vi "search for available lvclass files.vi"(6 "Folders to Exclude":string[](array[string]), 8 "error in":errorcluster, 11 "Plugin Search Paths":path[](array[path])) -> (0 "error out":errorcluster, 3 "discovered classes":path[](array[path]))   [LabVIEW 2013, in "class discovery singleton.lvlib"]
doc: "Finds all lvclass files, even inside llb and lvlibp files. Removes any in a folder titled \"\\builds\\\"."
uses:
  class discovery singleton.lvlib
  <vilib>/Utility/LVLibp/NI_PackedLibraryUtility.lvlib
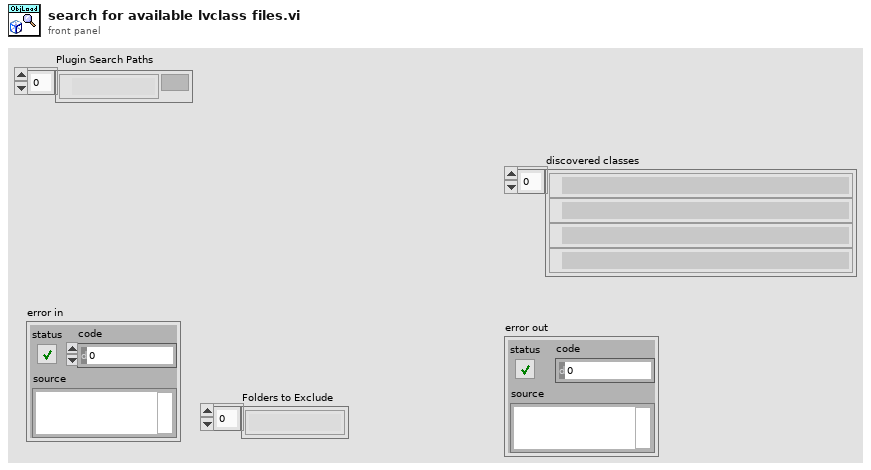
[diagram p1: front panel]
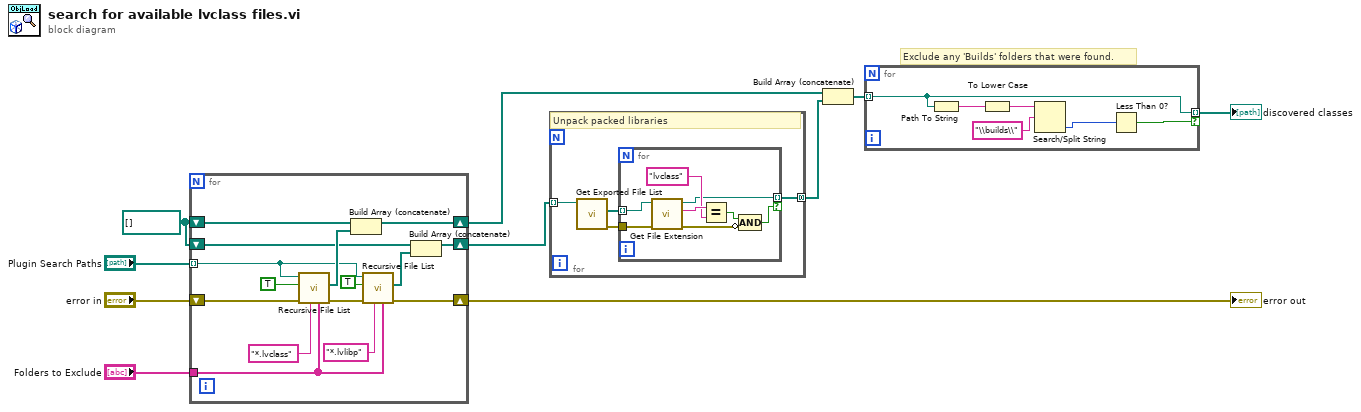
[diagram p0: block diagram]
diagram:
  w4 = path[] [] ("All Files in Dir")
  # "Exclude any 'Builds' folders that were found."
  n1 = for {
    tunnel: "Folders to Exclude" -> [w25]
    shift-right: [w15] -> w6
    shift-left: w4 -> [w16]
    shift-right: [w12] -> w8
    shift-left: w4 -> [w14]
    shift-right: [w19] -> w2
    shift-left: "error in" -> [w18]
    tunnel: "Plugin Search Paths" -> [w11] mode=indexing
    n2 = call <vilib>:"Recursive File List.vi"("Folders to Exclude"=w25, "pattern"="*.lvclass", "error in (no error)"=w18, "Treat LLBs as Folders?"=TRUE, "Folder Path"=w11) -> ("error out"=w22:errorcluster, "All Files in Dir"=w17:path[])  [unwired: 2 in, 3 out]
    n3 = Build Array (concatenate)(w16, w17) -> (w15:path[])
    n4 = call <vilib>:"Recursive File List.vi"("Folders to Exclude"=w25, "pattern"="*.lvlibp", "error in (no error)"=w22, "Treat LLBs as Folders?"=TRUE, "Folder Path"=w11) -> ("error out"=w19:errorcluster, "All Files in Dir"=w13:path[])  [unwired: 2 in, 3 out]
    n5 = Build Array (concatenate)(w14, w13) -> (w12:path[])
  }
  "error out" <- w2
  n6 = for {
    tunnel: w8 -> [w29] mode=indexing
    tunnel: [w26] -> w9 mode=concatenating
    # "Unpack packed libraries"
    n7 = call <vilib>:"Get Exported File List.vi"("packed library path"=w29) -> ("error out"=w28:errorcluster, "paths"=w27:path[])  [unwired: 8 in, 1 out]
    n8 = for {
      tunnel: w28 -> [w37]
      tunnel: w27 -> [w36] mode=indexing
      tunnel: [w31] -> w26 mode=indexing if=w30
      n9 = call <vilib>:"Get File Extension.vi"("error in (no error)"=w37, "file"=w36) -> ("error out"=w35:errorcluster, "lowercase file extension"=w33:string, "dup file"=w31:path)  [unwired: 6 in, 1 out]
      n10 = Equal?(x=w33, y="lvclass" ("x")) -> (x = y?=w34:bool)
      n11 = Compound Arithmetic op=AND(w34, invert w35) -> (w30:bool)
    }
  }
  n12 = Build Array (concatenate)(w6, w9) -> (w10:path[])
  n13 = for {
    tunnel: w10 -> [w40] mode=indexing
    tunnel: [w40] -> w1 mode=indexing if=w39
    n14 = Path To String(path=w40) -> (string=w43:string)
    n15 = To Lower Case(string=w43) -> (all lower case string=w42:string)
    n16 = Search/Split String(string=w42, search string/char (-)="\\builds\\") -> (offset of match=w38:i32)  [unwired: 1 in, 2 out]
    n17 = Less Than 0?(x=w38) -> (x < 0?=w39:bool)
  }
  "discovered classes" <- w1
